vi "myRIO_BRig_RT__Case_Exp_subState_LC.vi"(0 "input_dataCurrent":u16[](array[numeric]), 1 "input_spout":enum16{"Left", "Right"}(ring), 3 "LC_Cue1_OnOff":bool, 4 "LC_Cue1_Probability":u16, 7 "LC_Cue1_Block":u16(slide) max=2 step=1 scale=0.0..2.0, 9 "LC_Cue1_Trial":u16(slide) max=2 step=1 scale=0.0..1.0) -> (16 "output_LC":bool)   [LabVIEW 2014]
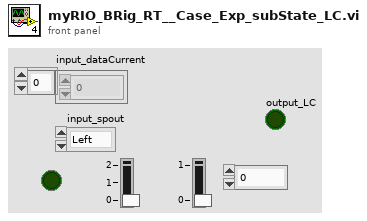
[diagram p1: front panel]
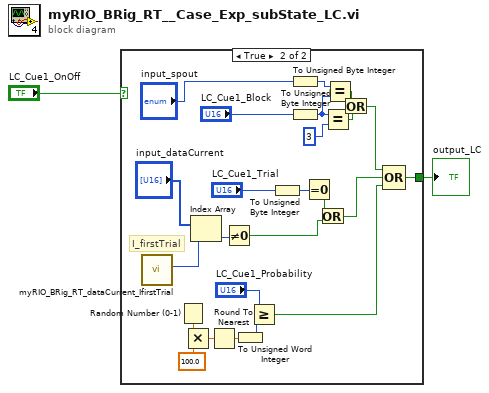
[diagram p0: block diagram]
diagram:
  n1 = case shown="True" "LC_Cue1_OnOff" {
    tunnel: [_ w8] -> w1
    frame False {
    }
    frame True {
      # "I_firstTrial"
      n2 = call "myRIO_BRig_RT_dataCurrent_IfirstTrial.vi"() -> ("output_I_firstTrial"=w20:i32)  [unwired: 11 in]
      n3 = Random Number (0-1)() -> (number: 0 to 1=w16:dbl)
      n4 = Multiply(x=w16, y=100.0) -> (x*y=w15:dbl)
      n5 = Index Array(array="input_dataCurrent", index=w20) -> (element=w19:u16)
      n6 = Round To Nearest(number=w15) -> (nearest integer value=w14:dbl)
      n7 = Not Equal To 0?(x=w19) -> (x != 0?=w17:bool)
      n8 = To Unsigned Word Integer(number=w14) -> (unsigned 16bit integer=w13:u16)
      n9 = Greater Or Equal?(x="LC_Cue1_Probability", y=w13) -> (x >= y?=w9:bool)
      n10 = To Unsigned Byte Integer(number="LC_Cue1_Trial") -> (unsigned 8bit integer=w21:u8)
      n11 = To Unsigned Byte Integer(number="input_spout") -> (unsigned 8bit integer=w25:u8)
      n12 = To Unsigned Byte Integer(number="LC_Cue1_Block") -> (unsigned 8bit integer=w24:u8)
      n13 = Equal To 0?(x=w21) -> (x = 0?=w18:bool)
      n14 = Or(x=w18, y=w17) -> (x .or. y?=w10:bool)
      n15 = Equal?(x=w24, y=u8 3) -> (x = y?=w22:bool)
      n16 = Equal?(x=w25, y=w24) -> (x = y?=w23:bool)
      n17 = Or(x=w23, y=w22) -> (x .or. y?=w11:bool)
      n18 = Compound Arithmetic op=OR(w11, w10, w9) -> (w8:bool)
    }
  }
  "output_LC" <- w1
